vi "Gestione coefficienti P2.vi"() -> (1 "Coefficenti P2 out":T1)   [LabVIEW 2019]
uses:
  <vilib>/Utility/file.llb/Write To Spreadsheet File (DBL).vi
  Globals.vi
  <vilib>/Utility/file.llb/Read From Spreadsheet File (DBL).vi
panel:
  out "selected path":path
  in  "Cluster P2":T2
  in  "Coefficenti P2":T1
  # "Freddo"
  # "Regime"
  # "Freddo"
  # "Regime"
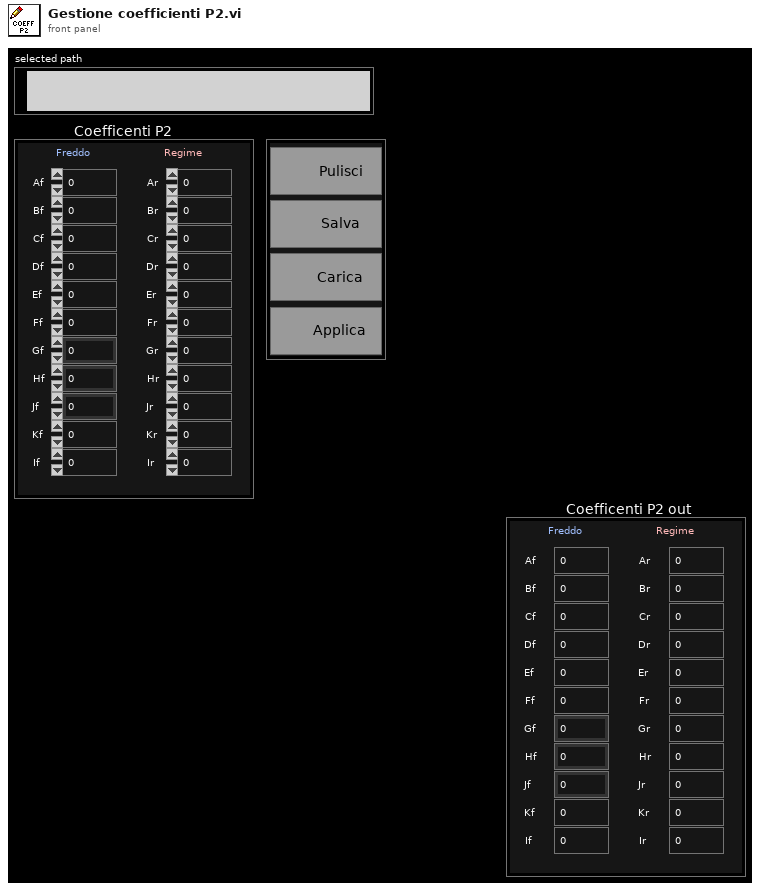
[diagram p1: front panel]
types:
  T1 = cluster{"Af":dbl, "Bf":dbl, "Cf":dbl, "Df":dbl, "Ef":dbl, "Ff":dbl, "Gf":dbl, "Hf":dbl, "Jf":dbl, "Kf":dbl, "If":dbl, "Ar":dbl, "Br":dbl, "Cr":dbl, "Dr":dbl, "Er":dbl, "Fr":dbl, "Gr":dbl, "Hr":dbl, "Jr":dbl, "Kr":dbl, "Ir":dbl}
  T2 = cluster{"APPLICA":bool, "SALVA":bool, "CARICA":bool, "APPLICA 2":bool}
  T3 = cluster{"Array of elements":cluster{"String":string, "variant":variant}[], "Single element":cluster{"String":string, "variant":variant}, "enque at\nopposite end (F)":bool, "no replications (F)":bool}
  T4 = cluster{"first row[0]":dbl, "first row[1]":dbl, "first row[2]":dbl, "first row[3]":dbl, "first row[4]":dbl, "first row[5]":dbl, "first row[6]":dbl, "first row[7]":dbl, "first row[8]":dbl, "first row[9]":dbl, "first row[10]":dbl, "first row[11]":dbl, "first row[12]":dbl, "first row[13]":dbl, "first row[14]":dbl, "first row[15]":dbl, "first row[16]":dbl, "first row[17]":dbl, "first row[18]":dbl, "first row[19]":dbl, "first row[20]":dbl, "first row[21]":dbl}
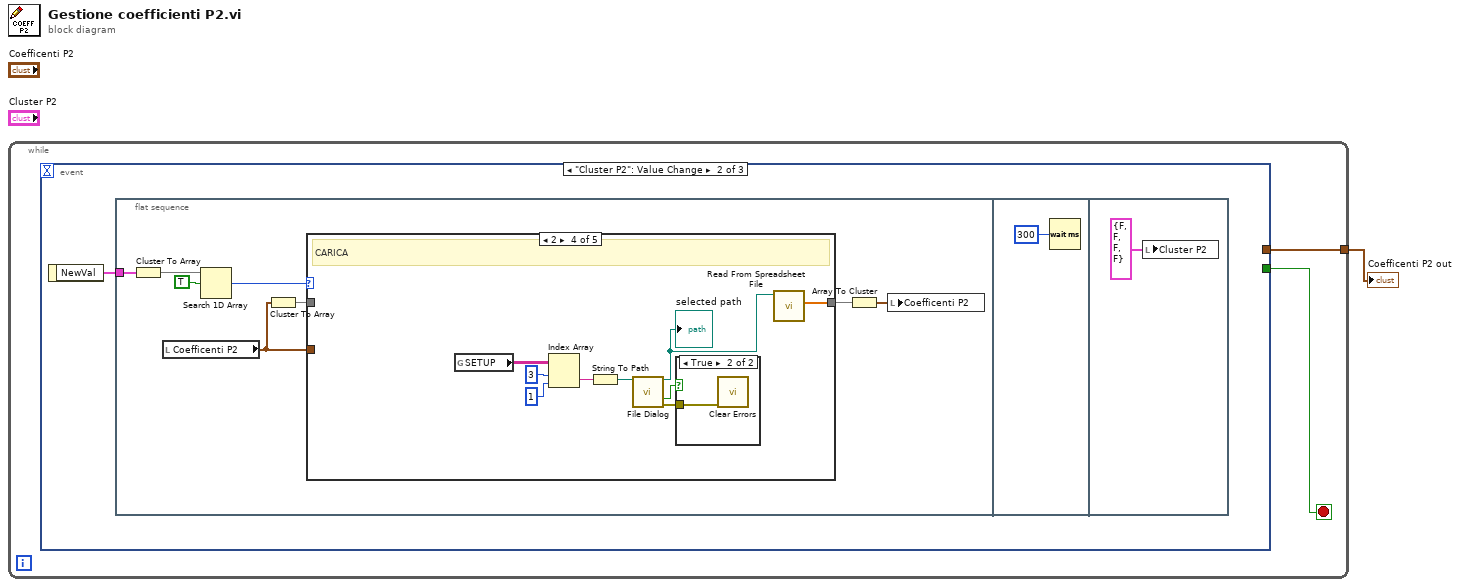
[diagram p0: block diagram]
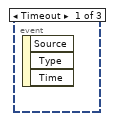
[diagram p2: hidden frame]
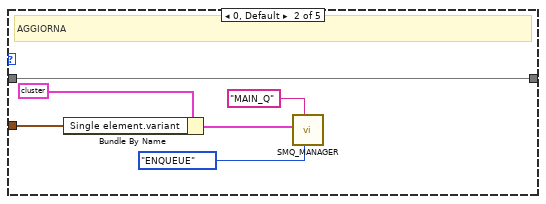
[diagram p4: hidden frame]
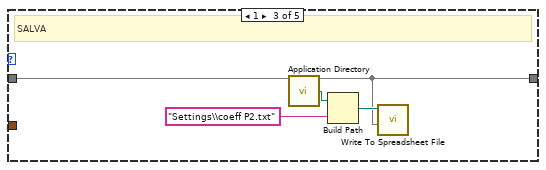
[diagram p5: hidden frame]
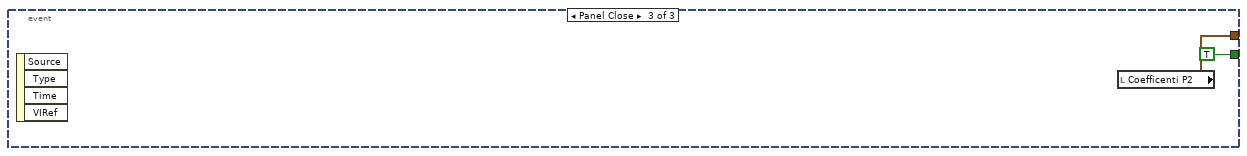
[diagram p8: hidden frame]
diagram:
  n1 = while {
    tunnel: [w2] -> w1
    stop <- w3 stop-if-true
    n2 = event shown="[1] \"Cluster P2\": Value Change" {
      selector: _ -> [_ _ _]
      dyn-events: _ -> [_ _ _]
      timeout: _ -> [_ _ _]
      tunnel: [_ _ TRUE] -> w3
      tunnel: [_ _ w36] -> w2
      event Timeout {
        n3 = event-data() -> ()  [unwired: 1 in, 3 out]
      }
      event "Cluster P2": Value Change {
        n4 = event-data() -> ("NewVal"=w4:T2)  [unwired: 1 in]
        n5 = flat-sequence {
          tunnel: w4 -> [w10]
          frame #0 {
            n6 = Cluster To Array(cluster=w10) -> (array=w11:bool[])
            n7 = local read "Coefficenti P2"() -> (w8:T1)
            n8 = Search 1D Array(1D array=w11, element=TRUE) -> (index of element=w9:i32)  [unwired: 1 in]
            n9 = Cluster To Array(cluster=w8) -> (array=w7:dbl[])
            n10 = case shown="2" w9 {
              tunnel: w7 -> [w13 w19 w20 _ _]
              tunnel: [w13 w19 w20 w32 _] -> w6
              tunnel: w8 -> [_ w14 _ _ _]
              frame -1 {
              }
              frame 0, Default {
                # "AGGIORNA"
                n11 = Bundle By Name(cluster=T3 {"Array of elements"=[], "Single element"={"String"="AGGIORNA COEFFICIENTI P2", "variant"=variant}, "enque at\nopposite end (F)"=FALSE, "no replications (F)"=FALSE} ("Enqueue cluster"), "Single element.variant"=w14) -> (w16:T3)
                n12 = call <userlib>:"SMQ_MANAGER.vi"("Function"=enum16{"INITIALIZE", "ENQUEUE", "STOP ALL"}."ENQUEUE", "Queue name"="MAIN_Q", "Enqueue cluster"=w16) -> ()  [unwired: 8 in, 1 out]
              }
              frame 1 {
                # "SALVA"
                n13 = call <vilib>:"Application Directory.vi"() -> ("Application Directory"=w23:path)
                n14 = Build Path(base path=w23, name or relative path="Settings\\coeff P2.txt") -> (appended path=w21:path)
                n15 = call-poly <vilib>:"Write To Spreadsheet File.vi"("1D data"=w20, "file path (dialog if empty)"=w21) -> ()  [unwired: 6 in, 1 out]
              }
              frame 2 {
                # "CARICA"
                n16 = global read "Globals.vi" "SETUP"() -> (w29:string[][])
                n17 = Index Array(array=w29, index (row)=3 ("disabled index (row)"), index (col)=1 ("disabled index (col)")) -> (element=w28:string)
                n18 = String To Path(string=w28) -> (path=w27:path)
                n19 = call "File Dialog"("start path"=w27) -> ("selected path"=w26:path, "cancelled"=w25:bool, "error out"=w24:errorcluster)  [unwired: 11 in, 1 out]
                "selected path" <- w26
                n20 = case shown="True" w25 {
                  tunnel: w24 -> [_ w33]
                  frame False {
                  }
                  frame True {
                    n21 = call <vilib>:"Clear Errors.vi"("error in (no error)"=w33) -> ()  [unwired: 5 in, 2 out]
                  }
                }
                n22 = call-poly <vilib>:"Read From Spreadsheet File.vi"("file path (dialog if empty)"=w26) -> ("first row"=w32:dbl[])  [unwired: 6 in, 4 out]
              }
              frame 3 {
                # "PULISCI"
              }
            }
            n23 = Array To Cluster(array=w6) -> (cluster=w5:T4)
            n24 = local write "Coefficenti P2"(w5) -> ()
          }
          frame #1 {
            n25 = Wait (ms)(milliseconds to wait=u32 300) -> ()  [unwired: 1 out]
          }
          frame #2 {
            n26 = local write "Cluster P2"(T2 {"APPLICA"=FALSE, "SALVA"=FALSE, "CARICA"=FALSE, "APPLICA 2"=FALSE} ("Cluster P2")) -> ()
          }
        }
      }
      event Panel Close {
        n27 = event-data() -> ()  [unwired: 1 in, 4 out]
        n28 = local read "Coefficenti P2"() -> (w36:T1)
      }
    }
  }
  "Coefficenti P2 out" <- w1
